vi "LW_MyVI_To_Select_Instrument.vi"(1 "Instrument Keys":string[](array[string]), 5 "error in (no error)":errorcluster) -> (15 "My Instrument Key":string, 19 "error out":errorcluster)   [LabVIEW 2010]
panel:
  in  "Continue":bool
  in  "Available Instrument Keys":u16(ring) items=["sample1", "sample2", "sample3"]
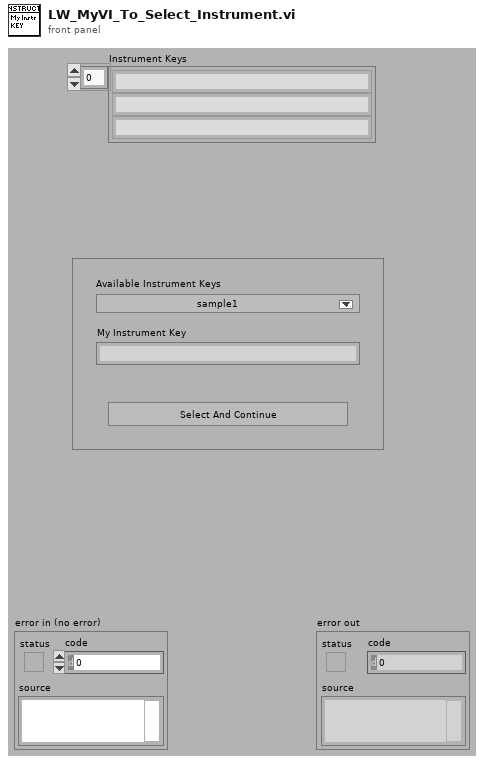
[diagram p1: front panel]
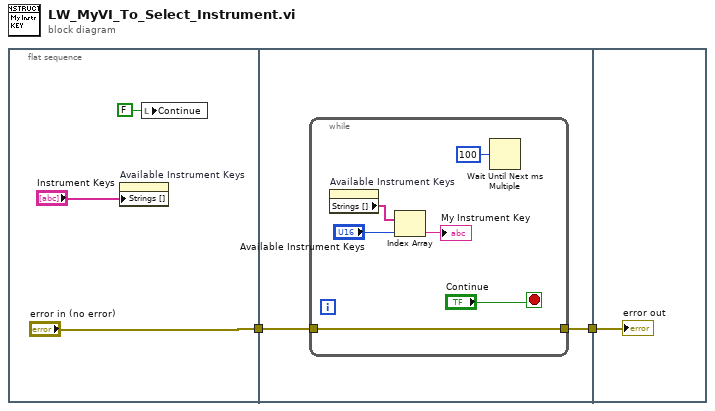
[diagram p0: block diagram]
diagram:
  n1 = flat-sequence {
    tunnel: ["error in (no error)"] -> w1
    tunnel: [w7] -> w2
    tunnel: w1 -> [w6]
    tunnel: w2 -> [w14]
    frame #0 {
      n2 = property on="Available Instrument Keys" class="Ring (strict)"("Strings []"="Instrument Keys") -> ()  [unwired: 2 in, 2 out]
      n3 = local write "Continue"(FALSE ("Continue")) -> ()
    }
    frame #1 {
      n4 = while {
        tunnel: [w8] -> w7
        tunnel: w6 -> [w8]
        stop <- "Continue" stop-if-true
        n5 = property on="Available Instrument Keys" class="Ring (strict)"() -> ("Strings []"=w11:string[])  [unwired: 2 in, 2 out]
        n6 = Index Array(array=w11, index="Available Instrument Keys") -> (element=→"My Instrument Key":string)
        n7 = Wait Until Next ms Multiple(millisecond multiple=u32 100) -> ()  [unwired: 1 out]
      }
    }
    frame #2 {
      "error out" <- w14
    }
  }
